vi "Path Edit.vi"() -> ()   [LabVIEW 2013]
uses:
  Global Variables.vi
panel:
  in  "Index":i32=8
  in  "Direction":u16(ring) items=["Forward", "Backward"]
  in  "Enabled":bool=TRUE
  in  "Voltage Schedule":u16(ring) items=["Constant", "Ramp", "Fn. Generator", "Formula"]
  in  "Apply to All":bool
  in  "Fill Orientation":u16(ring) items=["Horizontal", "Vertical"]
  in  "Smooth Segments":dbl=12.0
  in  "Speed Schedule":u16(ring) items=["Constant", "Ramp", "Fn. Generator", "Formula"]
  in  "Speed (µm/s)":dbl=8.0
  in  "Voltage (V)":dbl=8.0
  in  "Speed Settings":bool
  in  "Voltage Settings":bool
  in  "Fill Spacing":dbl=0.1
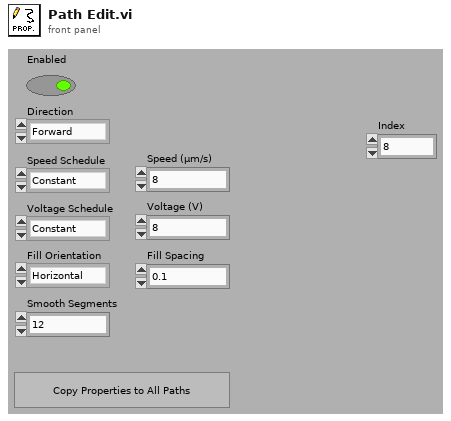
[diagram p1: front panel]
types:
  T1 = enum32{"invalid app kind", "Development System", "Run Time System", "Student Edition", "Embedded LabVIEW", "Evaluation", "Custom"}
  T2 = enum32{"Invalid", "Standard", "Closed", "Hidden", "Minimized", "Maximized"}
  T3 = cluster{"Enabled":bool, "Direction":u16, "Fill Orientation":u16, "Smooth Segments":dbl, "Fill Spacing":dbl, "Speed (µm/s)":cluster{"Schedule":u16, "Value":dbl, "Start Value":dbl, "End Value":dbl, "Min Value":dbl, "Max Value":dbl, "Duty Cycle (%)":dbl, "Signal Type":u16, "Cycle Number":dbl, "Phase (degrees)":dbl}, "Voltage (V)":cluster{"Schedule":u16, "Value":dbl, "Start Value":dbl, "End Value":dbl, "Min Value":dbl, "Max Value":dbl, "Duty Cycle (%)":dbl, "Signal Type":u16, "Cycle Number":dbl, "Phase (degrees)":dbl}}[]
  T4 = cluster{"Enabled":bool, "Direction":u16, "Fill Orientation":u16, "Smooth Segments":dbl, "Fill Spacing":dbl, "Speed (µm/s)":cluster{"Schedule":u16, "Value":dbl, "Start Value":dbl, "End Value":dbl, "Min Value":dbl, "Max Value":dbl, "Duty Cycle (%)":dbl, "Signal Type":u16, "Cycle Number":dbl, "Phase (degrees)":dbl}, "Voltage (V)":cluster{"Schedule":u16, "Value":dbl, "Start Value":dbl, "End Value":dbl, "Min Value":dbl, "Max Value":dbl, "Duty Cycle (%)":dbl, "Signal Type":u16, "Cycle Number":dbl, "Phase (degrees)":dbl}}
  T5 = cluster{"Schedule":u16, "Value":dbl, "Start Value":dbl, "End Value":dbl, "Min Value":dbl, "Max Value":dbl, "Duty Cycle (%)":dbl, "Signal Type":u16, "Cycle Number":dbl, "Phase (degrees)":dbl}
  T6 = cluster{"Schedule":u16, "Value":dbl, "Start Value":dbl, "End Value":dbl, "Min Value":dbl, "Max Value":dbl, "Duty Cycle (%)":dbl, "Speed Signal Type":u16, "Cycle Number":dbl, "Phase (degrees)":dbl}
  T7 = cluster{"Core":cluster{"Current VI Reference":refnum<vi>, "Close Panel on Exit?":bool}}
  T8 = cluster{"Current VI Reference":refnum<vi>, "Close Panel on Exit?":bool}
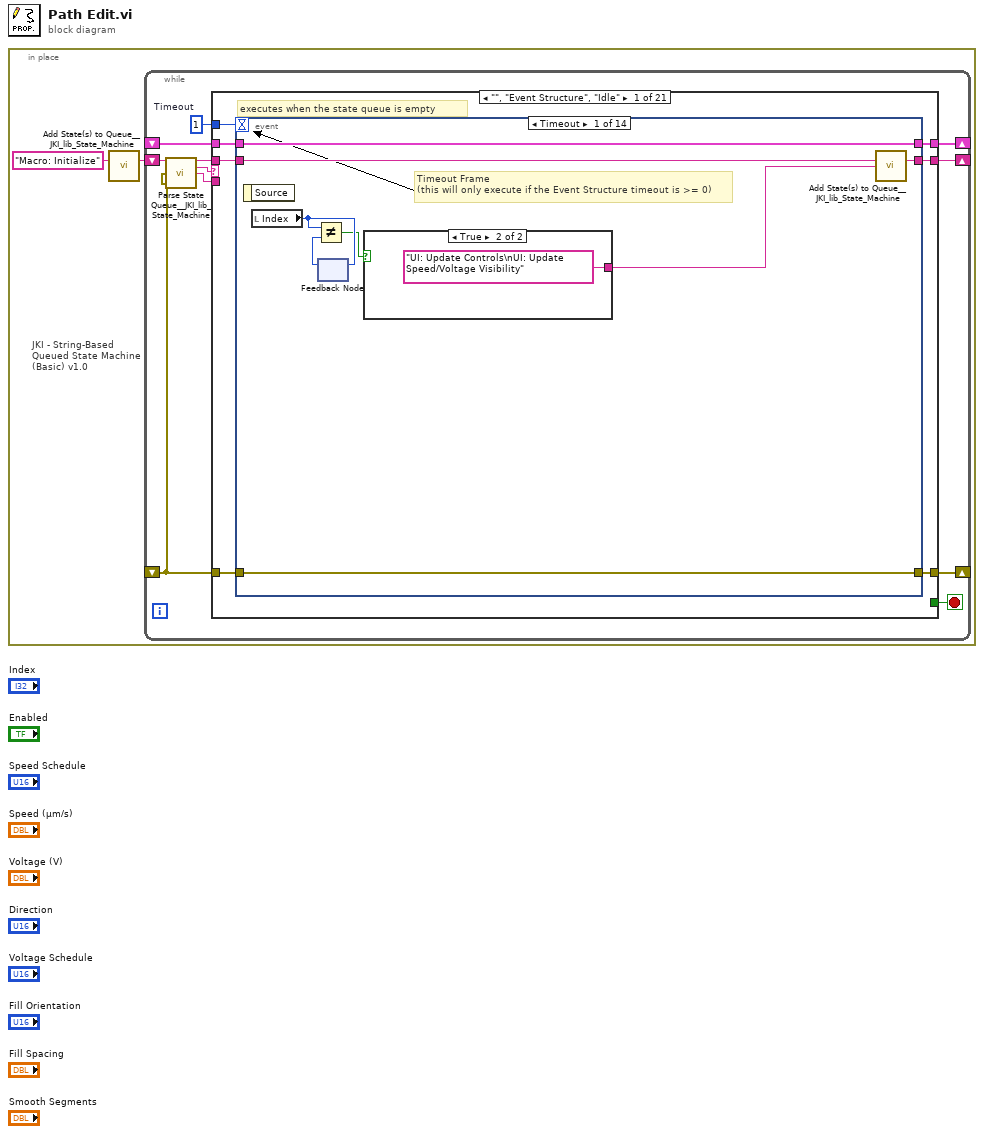
[diagram p0: block diagram]
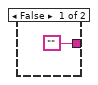
[diagram p2: hidden frame]
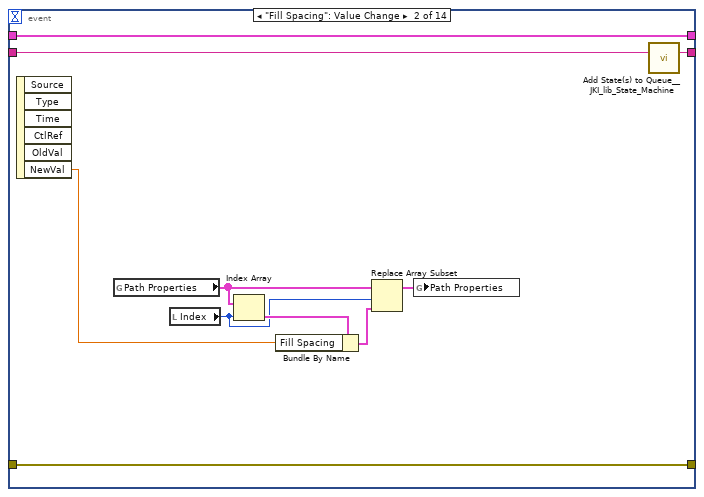
[diagram p3: hidden frame]
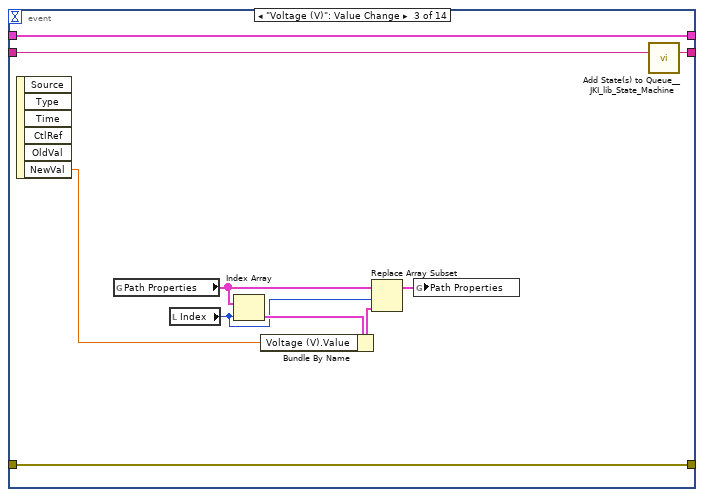
[diagram p4: hidden frame]
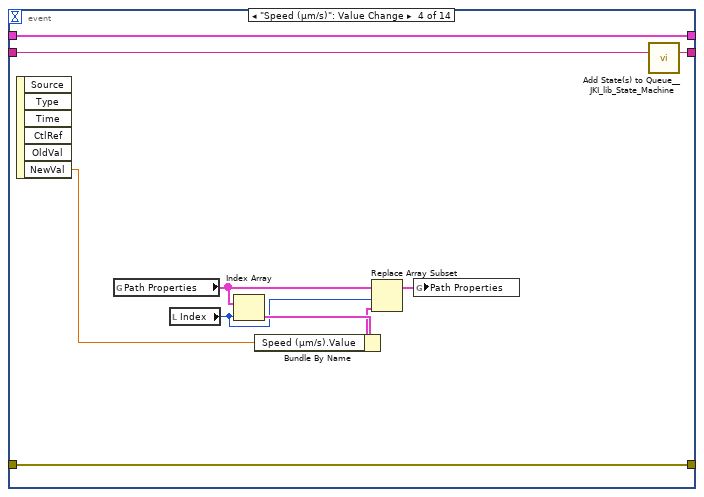
[diagram p5: hidden frame]
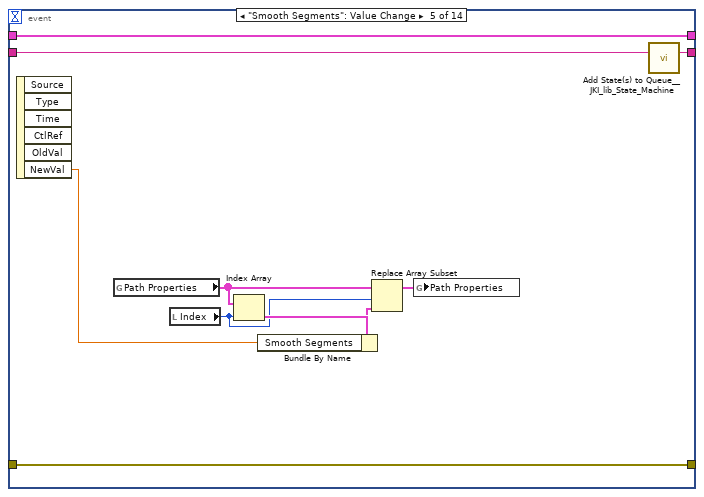
[diagram p6: hidden frame]
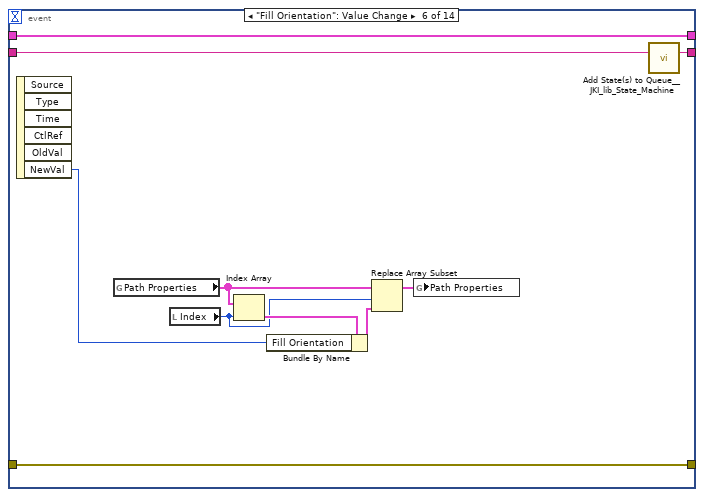
[diagram p7: hidden frame]
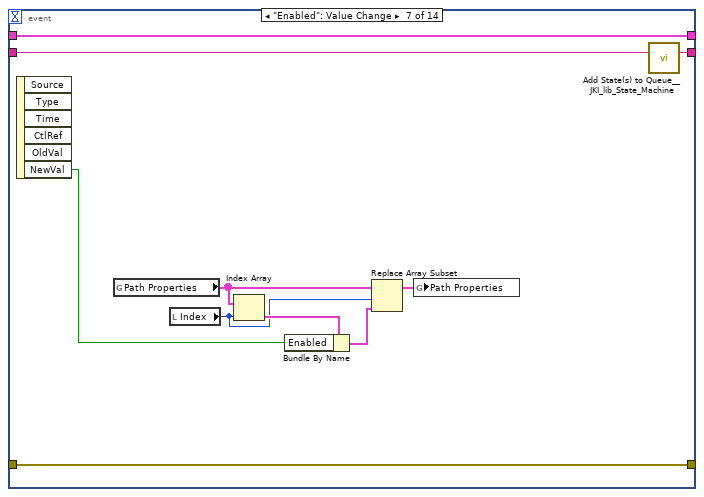
[diagram p8: hidden frame]
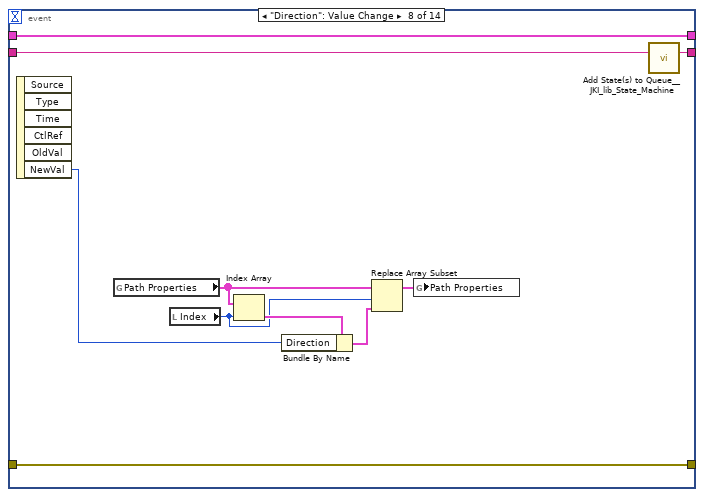
[diagram p9: hidden frame]
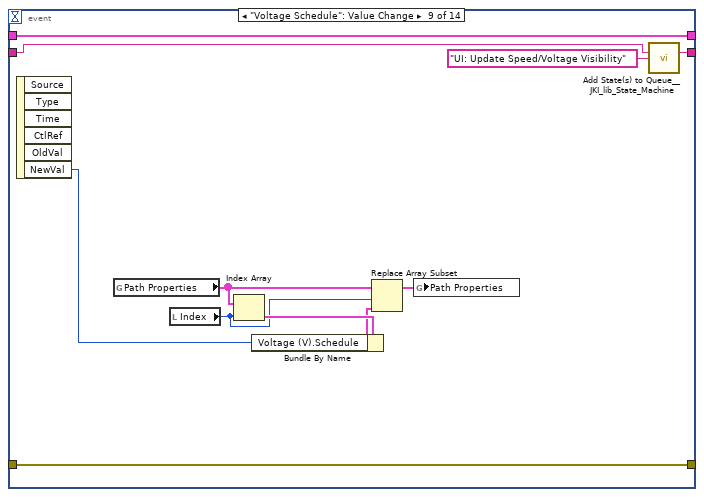
[diagram p10: hidden frame]
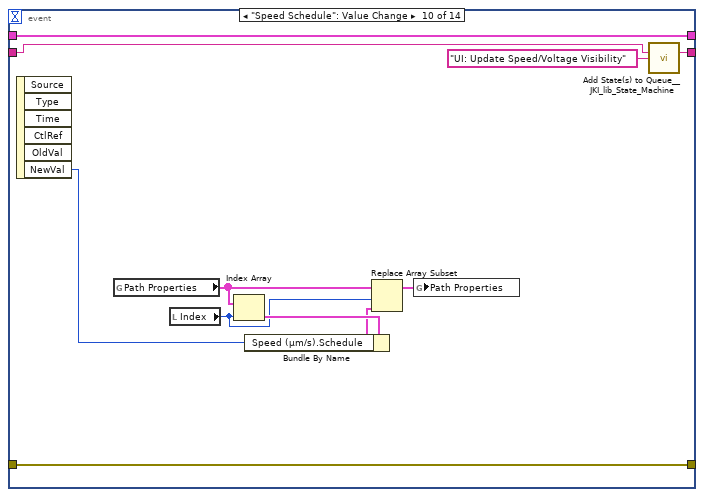
[diagram p11: hidden frame]
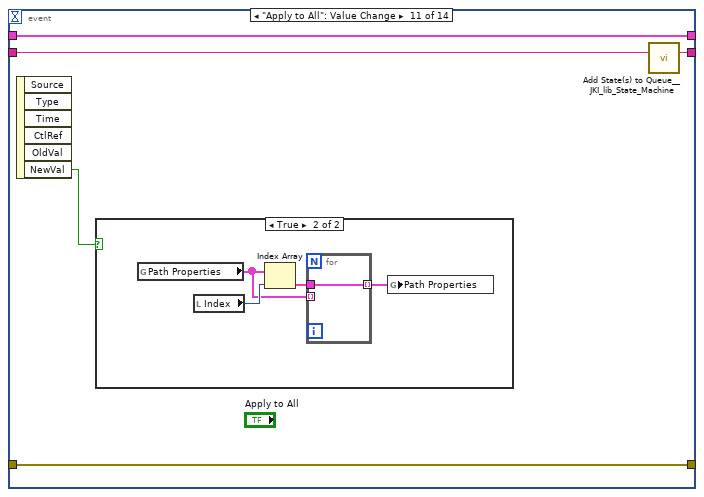
[diagram p12: hidden frame]
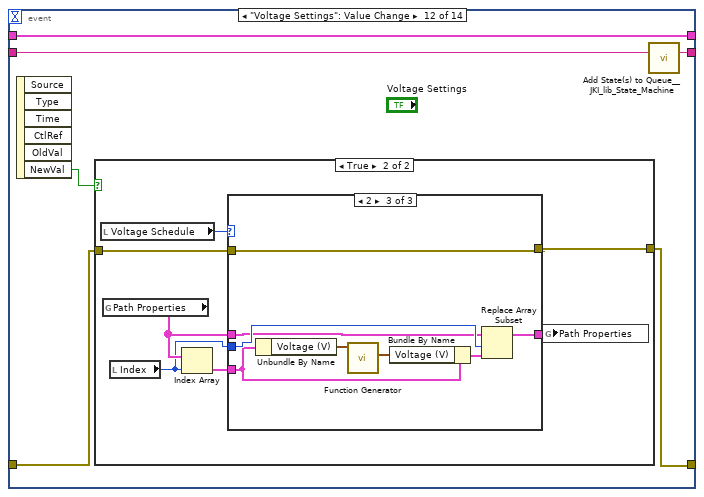
[diagram p14: hidden frame]
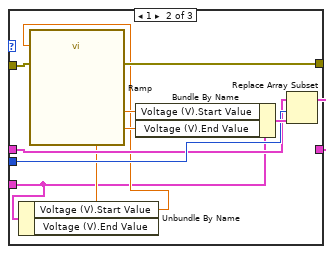
[diagram p17: hidden frame]
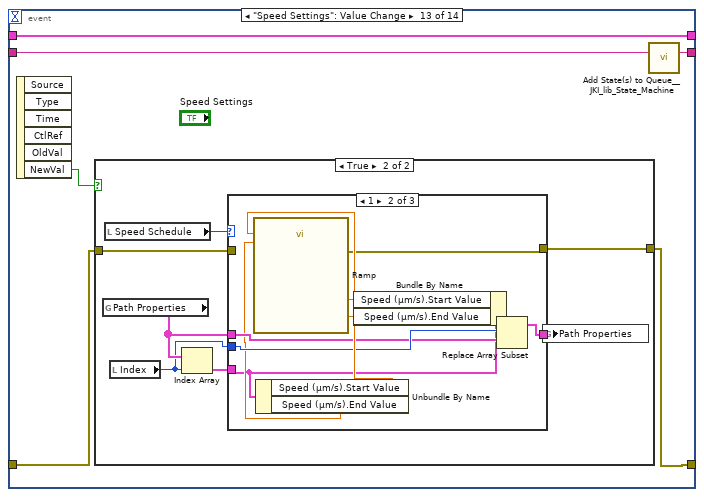
[diagram p18: hidden frame]
diagram:
  n1 = in-place {
    n2 = call <vilib>:"Add State(s) to Queue__JKI_lib_State_Machine.vi"("State(s) in (\"\")"="Macro: Initialize") -> ("States Out"=w2:string)  [unwired: 14 in]
    n3 = while "JKI - String-Based Queued State Machine (Basic) v1.0" {
      shift-right: [w6] -> _
      shift-left: _ -> [w5]
      shift-right: [w9] -> _
      shift-left: _ -> [w3]
      shift-right: [w8] -> _
      shift-left: w2 -> [w10]
      stop <- w7 stop-if-true
      w4 = 1  # Timeout
      n4 = call <vilib>:"Parse State Queue__JKI_lib_State_Machine.vi"("State Queue"=w10, "Error In (no error)"=w3) -> ("Remaining States"=w12:string, "Current State"=w13:string, "Arguments"=w11:string)  [unwired: 11 in]
      n5 = case shown="\"\", \"Event Structure\", \"Idle\"" w13 {
        selector: w13 -> [_ _ w212 _ _ _ _ _ _ _ _ _ _ _ _ _ _ _ _ _ _]
        tunnel: w12 -> [w20 w211 w216 w234 w240 w245 w249 w254 w260 w264 w268 w284 w290 w308 w319 w345 w350 w360 w364 w368 w372]
        tunnel: w11 -> [_ _ _ _ _ _ _ _ _ _ _ _ w285 _ w313 _ _ _ _ _ _]
        tunnel: w5 -> [w18 w208 w214 w230 w237 w243 w246 _ w258 w261 w266 w282 w288 w306 w315 w342 w347 w357 w361 w365 w369]
        tunnel: [w17 w209 w218 w231 errorcluster {"status"=FALSE, "code"=0, "source"=""} ("error out") w242 w247 w250 w256 w262 w265 w281 w286 w295 w316 w343 w348 w358 w362 w366 w370] -> w9
        tunnel: w3 -> [w16 w209 w217 w231 w236 w242 w247 w250 w255 w262 w265 w281 w287 w305 w317 w343 w348 w358 w362 w366 w370]
        tunnel: [w19 w210 w215 w233 w239 w244 w248 w253 w259 w263 w267 w283 w289 w307 w318 w344 w349 w359 w363 w367 w371] -> w8
        tunnel: [_ _ _ _ _ TRUE _ _ _ _ _ _ _ _ _ _ _ _ _ _ _] -> w7
        tunnel: [w15 w208 w214 w232 w237 w243 w246 w252 w258 w261 w266 w282 w288 w306 w315 w342 w347 w357 w361 w365 w369] -> w6
        tunnel: w4 -> [w14 _ _ _ _ _ _ _ _ _ _ _ _ _ _ _ _ _ _ _ _]
        frame "", "Event Structure", "Idle" {
          # "executes when the state queue is empty"
          n6 = event shown="[0] Timeout" {
            selector: _ -> [_ _ _ _ _ _ _ _ _ _ _ _ _ _]
            dyn-events: _ -> [_ _ _ _ _ _ _ _ _ _ _ _ _ _]
            timeout: w14 -> [_ _ _ _ _ _ _ _ _ _ _ _ _ _]
            tunnel: w20 -> [w28 w40 w50 w60 w70 w80 w90 w100 w111 w122 w127 w138 w173 w207]
            tunnel: [w27 w39 w49 w59 w69 w79 w89 w99 w110 w121 w126 w137 w172 w206] -> w19
            tunnel: w18 -> [w25 w38 w48 w58 w68 w78 w88 w98 w109 w120 w125 w136 w171 w204]
            tunnel: [w26 w32 w42 w52 w62 w72 w82 w92 w103 w114 w124 w134 w169 w205] -> w17
            tunnel: w16 -> [w26 w32 w42 w52 w62 w72 w82 w92 w103 w114 w124 w135 w170 w205]
            tunnel: [w25 w38 w48 w58 w68 w78 w88 w98 w109 w120 w125 w136 w171 w204] -> w15
            event Timeout {
              # "Timeout Frame\n(this will only execute if the Event Structure timeout is >= 0)"
              n7 = event-data() -> ()  [unwired: 1 in, 1 out]
              n8 = local read "Index"() -> (w23:i32)
              n9 = feedback #1() -> (w24:i32)  [unwired: 1 in]
              n10 = Not Equal?(x=w23, y=w24) -> (x != y?=w22:bool)
              n11 = feedback-in #1(w23) -> ()
              n12 = case shown="True" w22 {
                tunnel: ["" "UI: Update Controls\nUI: Update Speed/Voltage Visibility"] -> w21
                frame False {
                }
                frame True {
                }
              }
              n13 = call <vilib>:"Add State(s) to Queue__JKI_lib_State_Machine.vi"("State(s) in (\"\")"=w28, "State(s) at Back (\"\")"=w21) -> ("States Out"=w27:string)  [unwired: 13 in]
            }
            event "Fill Spacing": Value Change {
              n14 = event-data() -> ("NewVal"=w36:dbl)  [unwired: 1 in, 5 out]
              n15 = global read "Global Variables.vi" "Path Properties"() -> (w34:T3)
              n16 = local read "Index"() -> (w31:i32)
              n17 = Index Array(array=w34, index=w31) -> (element=w37:T4)
              n18 = Bundle By Name(cluster=w37, "Fill Spacing"=w36) -> (w35:T4)
              n19 = Replace Array Subset(array=w34, new element=w35, index=w31) -> (w33:T3)
              n20 = global write "Global Variables.vi" "Path Properties"(w33) -> ()
              n21 = call <vilib>:"Add State(s) to Queue__JKI_lib_State_Machine.vi"("State(s) in (\"\")"=w40) -> ("States Out"=w39:string)  [unwired: 14 in]
            }
            event "Voltage (V)": Value Change {
              n22 = event-data() -> ("NewVal"=w46:dbl)  [unwired: 1 in, 5 out]
              n23 = global read "Global Variables.vi" "Path Properties"() -> (w44:T3)
              n24 = local read "Index"() -> (w41:i32)
              n25 = Index Array(array=w44, index=w41) -> (element=w47:T4)
              n26 = Bundle By Name(cluster=w47, "Voltage (V).Value"=w46) -> (w45:T4)
              n27 = Replace Array Subset(array=w44, new element=w45, index=w41) -> (w43:T3)
              n28 = global write "Global Variables.vi" "Path Properties"(w43) -> ()
              n29 = call <vilib>:"Add State(s) to Queue__JKI_lib_State_Machine.vi"("State(s) in (\"\")"=w50) -> ("States Out"=w49:string)  [unwired: 14 in]
            }
            event "Speed (µm/s)": Value Change {
              n30 = event-data() -> ("NewVal"=w56:dbl)  [unwired: 1 in, 5 out]
              n31 = global read "Global Variables.vi" "Path Properties"() -> (w54:T3)
              n32 = local read "Index"() -> (w51:i32)
              n33 = Index Array(array=w54, index=w51) -> (element=w57:T4)
              n34 = Bundle By Name(cluster=w57, "Speed (µm/s).Value"=w56) -> (w55:T4)
              n35 = Replace Array Subset(array=w54, new element=w55, index=w51) -> (w53:T3)
              n36 = global write "Global Variables.vi" "Path Properties"(w53) -> ()
              n37 = call <vilib>:"Add State(s) to Queue__JKI_lib_State_Machine.vi"("State(s) in (\"\")"=w60) -> ("States Out"=w59:string)  [unwired: 14 in]
            }
            event "Smooth Segments": Value Change {
              n38 = event-data() -> ("NewVal"=w66:dbl)  [unwired: 1 in, 5 out]
              n39 = global read "Global Variables.vi" "Path Properties"() -> (w64:T3)
              n40 = local read "Index"() -> (w61:i32)
              n41 = Index Array(array=w64, index=w61) -> (element=w67:T4)
              n42 = Bundle By Name(cluster=w67, "Smooth Segments"=w66) -> (w65:T4)
              n43 = Replace Array Subset(array=w64, new element=w65, index=w61) -> (w63:T3)
              n44 = global write "Global Variables.vi" "Path Properties"(w63) -> ()
              n45 = call <vilib>:"Add State(s) to Queue__JKI_lib_State_Machine.vi"("State(s) in (\"\")"=w70) -> ("States Out"=w69:string)  [unwired: 14 in]
            }
            event "Fill Orientation": Value Change {
              n46 = event-data() -> ("NewVal"=w76:u16)  [unwired: 1 in, 5 out]
              n47 = global read "Global Variables.vi" "Path Properties"() -> (w74:T3)
              n48 = local read "Index"() -> (w71:i32)
              n49 = Index Array(array=w74, index=w71) -> (element=w77:T4)
              n50 = Bundle By Name(cluster=w77, "Fill Orientation"=w76) -> (w75:T4)
              n51 = Replace Array Subset(array=w74, new element=w75, index=w71) -> (w73:T3)
              n52 = global write "Global Variables.vi" "Path Properties"(w73) -> ()
              n53 = call <vilib>:"Add State(s) to Queue__JKI_lib_State_Machine.vi"("State(s) in (\"\")"=w80) -> ("States Out"=w79:string)  [unwired: 14 in]
            }
            event "Enabled": Value Change {
              n54 = event-data() -> ("NewVal"=w86:bool)  [unwired: 1 in, 5 out]
              n55 = global read "Global Variables.vi" "Path Properties"() -> (w84:T3)
              n56 = local read "Index"() -> (w81:i32)
              n57 = Index Array(array=w84, index=w81) -> (element=w87:T4)
              n58 = Bundle By Name(cluster=w87, "Enabled"=w86) -> (w85:T4)
              n59 = Replace Array Subset(array=w84, new element=w85, index=w81) -> (w83:T3)
              n60 = global write "Global Variables.vi" "Path Properties"(w83) -> ()
              n61 = call <vilib>:"Add State(s) to Queue__JKI_lib_State_Machine.vi"("State(s) in (\"\")"=w90) -> ("States Out"=w89:string)  [unwired: 14 in]
            }
            event "Direction": Value Change {
              n62 = event-data() -> ("NewVal"=w96:u16)  [unwired: 1 in, 5 out]
              n63 = global read "Global Variables.vi" "Path Properties"() -> (w94:T3)
              n64 = local read "Index"() -> (w91:i32)
              n65 = Index Array(array=w94, index=w91) -> (element=w97:T4)
              n66 = Bundle By Name(cluster=w97, "Direction"=w96) -> (w95:T4)
              n67 = Replace Array Subset(array=w94, new element=w95, index=w91) -> (w93:T3)
              n68 = global write "Global Variables.vi" "Path Properties"(w93) -> ()
              n69 = call <vilib>:"Add State(s) to Queue__JKI_lib_State_Machine.vi"("State(s) in (\"\")"=w100) -> ("States Out"=w99:string)  [unwired: 14 in]
            }
            event "Voltage Schedule": Value Change {
              n70 = event-data() -> ("NewVal"=w107:u16)  [unwired: 1 in, 5 out]
              n71 = global read "Global Variables.vi" "Path Properties"() -> (w105:T3)
              n72 = local read "Index"() -> (w101:i32)
              n73 = Index Array(array=w105, index=w101) -> (element=w108:T4)
              n74 = Bundle By Name(cluster=w108, "Voltage (V).Schedule"=w107) -> (w106:T4)
              n75 = Replace Array Subset(array=w105, new element=w106, index=w101) -> (w104:T3)
              n76 = global write "Global Variables.vi" "Path Properties"(w104) -> ()
              n77 = call <vilib>:"Add State(s) to Queue__JKI_lib_State_Machine.vi"("State(s) in (\"\")"=w111, "State(s) at Back (\"\")"="UI: Update Speed/Voltage Visibility" ("State(s) at Back (\"\")")) -> ("States Out"=w110:string)  [unwired: 13 in]
            }
            event "Speed Schedule": Value Change {
              n78 = event-data() -> ("NewVal"=w118:u16)  [unwired: 1 in, 5 out]
              n79 = global read "Global Variables.vi" "Path Properties"() -> (w116:T3)
              n80 = local read "Index"() -> (w112:i32)
              n81 = Index Array(array=w116, index=w112) -> (element=w119:T4)
              n82 = Bundle By Name(cluster=w119, "Speed (µm/s).Schedule"=w118) -> (w117:T4)
              n83 = Replace Array Subset(array=w116, new element=w117, index=w112) -> (w115:T3)
              n84 = global write "Global Variables.vi" "Path Properties"(w115) -> ()
              n85 = call <vilib>:"Add State(s) to Queue__JKI_lib_State_Machine.vi"("State(s) in (\"\")"=w122, "State(s) at Back (\"\")"="UI: Update Speed/Voltage Visibility" ("State(s) at Back (\"\")")) -> ("States Out"=w121:string)  [unwired: 13 in]
            }
            event "Apply to All": Value Change {
              n86 = event-data() -> ("NewVal"=w123:bool)  [unwired: 1 in, 5 out]
              n87 = case shown="True" w123 {
                frame False {
                }
                frame True {
                  n88 = global read "Global Variables.vi" "Path Properties"() -> (w128:T3)
                  n89 = local read "Index"() -> (w131:i32)
                  n90 = Index Array(array=w128, index=w131) -> (element=w130:T4)
                  n91 = for {
                    tunnel: w130 -> [w132]
                    tunnel: [w132] -> w129 mode=indexing
                    tunnel: w128 -> [_] mode=indexing
                  }
                  n92 = global write "Global Variables.vi" "Path Properties"(w129) -> ()
                }
              }
              n93 = call <vilib>:"Add State(s) to Queue__JKI_lib_State_Machine.vi"("State(s) in (\"\")"=w127) -> ("States Out"=w126:string)  [unwired: 14 in]
            }
            event "Voltage Settings": Value Change {
              n94 = event-data() -> ("NewVal"=w133:bool)  [unwired: 1 in, 5 out]
              n95 = case shown="True" w133 {
                tunnel: w135 -> [w139 w145]
                tunnel: [w139 w144] -> w134
                frame False {
                }
                frame True {
                  n96 = local read "Voltage Schedule"() -> (w146:u16)
                  n97 = global read "Global Variables.vi" "Path Properties"() -> (w141:T3)
                  n98 = local read "Index"() -> (w140:i32)
                  n99 = Index Array(array=w141, index=w140) -> (element=w142:T4)
                  n100 = case shown="2" w146 {
                    tunnel: w145 -> [w148 w159 w163]
                    tunnel: [w148 w152 w163] -> w144
                    tunnel: [w147 w153 w164] -> w143
                    tunnel: w142 -> [_ w149 w162]
                    tunnel: w141 -> [w147 w154 w165]
                    tunnel: w140 -> [_ w155 w166]
                    frame 0, Default {
                    }
                    frame 1 {
                      n101 = Unbundle By Name(w149) -> ("Voltage (V).Start Value"=w151:dbl, "Voltage (V).End Value"=w150:dbl)
                      n102 = call "Ramp.vi"("Start Value"=w151, "End Value"=w150, "error in (no error)"=w159) -> ("End Value"=w157:dbl, "Start Value"=w158:dbl, "error out"=w152:errorcluster)  [unwired: 13 in, 1 out]
                      n103 = Bundle By Name(cluster=w149, "Voltage (V).Start Value"=w158, "Voltage (V).End Value"=w157) -> (w156:T4)
                      n104 = Replace Array Subset(array=w154, new element=w156, index=w155) -> (w153:T3)
                    }
                    frame 2 {
                      n105 = Unbundle By Name(w162) -> ("Voltage (V)"=w160:T5)
                      n106 = call "Function Generator.vi"("Properties in"=w160) -> ("Properties out"=w161:T6)  [unwired: 9 in, 1 out]
                      n107 = Bundle By Name(cluster=w162, "Voltage (V)"=w161) -> (w167:T4)
                      n108 = Replace Array Subset(array=w165, new element=w167, index=w166) -> (w164:T3)
                    }
                  }
                  n109 = global write "Global Variables.vi" "Path Properties"(w143) -> ()
                }
              }
              n110 = call <vilib>:"Add State(s) to Queue__JKI_lib_State_Machine.vi"("State(s) in (\"\")"=w138) -> ("States Out"=w137:string)  [unwired: 14 in]
            }
            event "Speed Settings": Value Change {
              n111 = event-data() -> ("NewVal"=w168:bool)  [unwired: 1 in, 5 out]
              n112 = case shown="True" w168 {
                tunnel: w170 -> [w174 w180]
                tunnel: [w174 w179] -> w169
                frame False {
                }
                frame True {
                  n113 = global read "Global Variables.vi" "Path Properties"() -> (w176:T3)
                  n114 = local read "Speed Schedule"() -> (w181:u16)
                  n115 = local read "Index"() -> (w175:i32)
                  n116 = Index Array(array=w176, index=w175) -> (element=w177:T4)
                  n117 = case shown="1" w181 {
                    tunnel: w180 -> [w183 _ w197]
                    tunnel: [w183 w189 w197] -> w179
                    tunnel: [w182 w188 w198] -> w178
                    tunnel: w177 -> [_ w184 w196]
                    tunnel: w176 -> [w182 w186 w199]
                    tunnel: w175 -> [_ w187 w200]
                    frame 0, Default {
                    }
                    frame 1 {
                      n118 = Unbundle By Name(w184) -> ("Speed (µm/s).Start Value"=w190:dbl, "Speed (µm/s).End Value"=w185:dbl)
                      n119 = call "Ramp.vi"("Start Value"=w190, "End Value"=w185) -> ("End Value"=w192:dbl, "Start Value"=w193:dbl, "error out"=w189:errorcluster)  [unwired: 14 in, 1 out]
                      n120 = Bundle By Name(cluster=w184, "Speed (µm/s).Start Value"=w193, "Speed (µm/s).End Value"=w192) -> (w191:T4)
                      n121 = Replace Array Subset(array=w186, new element=w191, index=w187) -> (w188:T3)
                    }
                    frame 2 {
                      n122 = Unbundle By Name(w196) -> ("Speed (µm/s)"=w194:T5)
                      n123 = call "Function Generator.vi"("Properties in"=w194) -> ("Properties out"=w195:T6)  [unwired: 9 in, 1 out]
                      n124 = Bundle By Name(cluster=w196, "Speed (µm/s)"=w195) -> (w201:T4)
                      n125 = Replace Array Subset(array=w199, new element=w201, index=w200) -> (w198:T3)
                    }
                  }
                  n126 = global write "Global Variables.vi" "Path Properties"(w178) -> ()
                }
              }
              n127 = call <vilib>:"Add State(s) to Queue__JKI_lib_State_Machine.vi"("State(s) in (\"\")"=w173) -> ("States Out"=w172:string)  [unwired: 14 in]
            }
            event Panel Close? {
              # "Discard the event because we'll close the front panel ourselves in Macro: Exit"
              # "Close Panel button (pressed) Event\n(this executes Macro: Exit to terminate the VI)"
              n128 = event-data() -> ()  [unwired: 1 in, 1 out]
              n129 = event-data("Discard?"=TRUE) -> ()  [unwired: 1 in, 1 out]
              n130 = call <vilib>:"Add State(s) to Queue__JKI_lib_State_Machine.vi"("State(s) in Front (\"\")"="Macro: Exit", "State(s) in (\"\")"=w207) -> ("States Out"=w206:string)  [unwired: 13 in]
            }
          }
        }
        frame "---------- Core ----------" {
          # "Do not put any code in this frame.\n(it is a separator no-op)"
          n131 = call <vilib>:"Add State(s) to Queue__JKI_lib_State_Machine.vi"("State(s) in (\"\")"=w211) -> ("States Out"=w210:string)  [unwired: 14 in]
        }
        frame Default {
          w221 = 42 items=["No error", "Argument error", "Memory is full", "Out of zone", "End of file", "File already open", "Generic file I/O error", "File not found", "File permission error", "Disk is full", "Duplicate path", "Too many files open", "System feature not enabled", "Resource file not found", "Cannot add resource", "Resource not found", "Image not found", "Image memory error", "Pen does not exist", "Config type invalid", "Config token not found", "Config parse error", "Config memory error", "Bad external code format", "Bad external code offset", "External code not present", "Null window", "Destroy window error", "Null menu", "Print aborted", "Bad print record", "Print driver error", "Windows error during printing", "Memory error during printing", "Print dialog error", "Generic print error", "Invalid device refnum", "Device not found", "Device parameter error", "Device unit error", "Cannot open device", "Device call aborted", "Generic error", "Cancelled by user", "Object ID too low", "Object ID too high", "Object not in heap", "Unknown heap", "Unknown object (invalid DefProc)", "Unknown object (DefProc not in table)", "Message out of range", "Invalid (null) method", "Unknown message", "Manager call not supported", "Bad address", "Network operation in progress", "Network operation timed out", "Connection is busy", "Network attribute not supported", "Network error", "Address in use", "System out of memory", "Connection aborted", "Connection refused", "Not connected", "Already connected", "Connection closed", "Initialization error (interapplication manager)", "Bad occurrence", "Wait on unbound occurrence handler", "Occurrence queue overflow", "Datalog type conflict", "Unused", "Unrecognized type (interapplication manager)", "Memory corrupt", "Failed to make temporary DLL", "Old CIN version", "Drag socket not found", "Failed to load drop-object", "Failed to register OLE object", "Failed to release OLE object", "Format specifier type mismatch", "Unknown format specifier", "Too few format specifiers", "Too many format specifiers", "Scan failed", "Newer CIN version", "Error converting to variant", "Runtime menu error", "Password tampered", "Variant attribute not found", "Incompatible variant data type", "Event data is not available", "Event Store is not present", "Occurrence is not found", "Event Queue is not created", "Event info is not available", "Refnum passed is NULL", "Error retrieving Class GUID", "Error retrieving CoClass GUID", "Error retrieving TypeLib GUID.", "Bad built application magic bytes.", "Specific driver is different from the specific driver associated with the Logical Name.", "There is no session opened to the class driver.", "Max Error", "MAX - Error with config objects", "MAX - Error loading configuration", "MAX - Group not supported"]
          # "Current State"
          # "Do not delete, rename, or modify this frame.\n(this is used to capture unhandled states and typos)"
          # "Handle mistyped state name (developer tool)"
          n132 = Format Into String(format string="Software Exception: Unhandled State \"%s\"." ("message"), error in=w217, w212) -> (resulting string=w220:string, error out=w219:errorcluster)  [unwired: 1 in]
          n133 = call <vilib>:"Error Cluster From Error Code.vi"("show call chain? (False)"=TRUE, "error in (no error)"=w219, "error message (\"\")"=w220, "error code (0)"=w221) -> ("error out"=w218:errorcluster)  [unwired: 5 in]
          n134 = call <vilib>:"Add State(s) to Queue__JKI_lib_State_Machine.vi"("State(s) in (\"\")"=w216) -> ("States Out"=w215:string)  [unwired: 14 in]
        }
        frame "Initialize Core Data" {
          # "exe?"
          # "If panel starts closed or is an EXE, then close it when we exit"
          # "Do not delete, rename, or modify this frame.\n(this is used to determine panel behavior on exit)"
          n135 = control-ref of="Current VI Reference"() -> (w229:refnum<vi>)
          n136 = property class="VI"() -> ("Front Panel.Open"=w228:bool)  [unwired: 2 in, 2 out]
          n137 = property class="App"() -> ("App.Kind"=w227:T1)  [unwired: 2 in, 2 out]
          n138 = Not(x=w228) -> (.not. x?=w225:bool)
          n139 = Equal?(x=w227, y=T1."Run Time System" ("Application:Kind")) -> (x = y?=w224:bool)
          n140 = Or(x=w225, y=w224) -> (x .or. y?=w223:bool)
          n141 = Bundle By Name(cluster=w230, "Core.Current VI Reference"=w229, "Core.Close Panel on Exit?"=w223) -> (w232:T7)
          n142 = call <vilib>:"Add State(s) to Queue__JKI_lib_State_Machine.vi"("State(s) in (\"\")"=w234) -> ("States Out"=w233:string)  [unwired: 14 in]
        }
        frame "Error Handler" {
          # "Unhandled Error -- Display it"
          # "Handle any errors here.\nYou can also output any states to clean-up after errors occur"
          # "Clear error"
          n143 = call <vilib>:"General Error Handler.vi"("error in (no error)"=w236) -> ()  [unwired: 10 in, 5 out]
          n144 = call <vilib>:"Add State(s) to Queue__JKI_lib_State_Machine.vi"("State(s) in Front (\"\")"="/* Post Error States", "State(s) in (\"\")"=w240) -> ("States Out"=w239:string)  [unwired: 13 in]
        }
        frame "Exit" {
          # "Do not put any code in this frame.\n(No errors that occur here will be handled.)"
          n145 = call <vilib>:"Add State(s) to Queue__JKI_lib_State_Machine.vi"("State(s) in (\"\")"=w245) -> ("States Out"=w244:string)  [unwired: 14 in]
        }
        frame "---------- Data ----------" {
          # "Do not put any code in this frame.\n(It is a separator no-op. You can make a copy of this frame to create a new Data frame)"
          n146 = call <vilib>:"Add State(s) to Queue__JKI_lib_State_Machine.vi"("State(s) in (\"\")"=w249) -> ("States Out"=w248:string)  [unwired: 14 in]
        }
        frame "Data: Initialize" {
          w251 = T8 {"Current VI Reference"=refnum, "Close Panel on Exit?"=FALSE}  # Core
          # "Initialize the shift-register data, here.\n(data names are defined by what you wire into the bundle function)"
          n147 = Bundle("Core"=w251) -> (w252:T7)  [unwired: 1 in]
          n148 = call <vilib>:"Add State(s) to Queue__JKI_lib_State_Machine.vi"("State(s) in (\"\")"=w254) -> ("States Out"=w253:string)  [unwired: 14 in]
        }
        frame "Data: Cleanup" {
          # "Cleanup any data and references, here.\n(this is called automatically, by the Macro: Exit)"
          n149 = Unbundle By Name(w258) -> ("Core.Current VI Reference"=w257:refnum<vi>)
          n150 = Close Reference(reference=w257, error in (no error)=w255) -> (error out=w256:errorcluster)
          n151 = call <vilib>:"Add State(s) to Queue__JKI_lib_State_Machine.vi"("State(s) in (\"\")"=w260) -> ("States Out"=w259:string)  [unwired: 14 in]
        }
        frame "---------- UI ----------" {
          # "Do not put any code in this frame.\n(It is a separator no-op. You can make a copy of this frame to create a new UI frame)"
          n152 = call <vilib>:"Add State(s) to Queue__JKI_lib_State_Machine.vi"("State(s) in (\"\")"=w264) -> ("States Out"=w263:string)  [unwired: 14 in]
        }
        frame "UI: Initialize" {
          # "Initialize the User Interface, here.\n(this is called automatically, by the Macro: Init)"
          n153 = call <vilib>:"Add State(s) to Queue__JKI_lib_State_Machine.vi"("State(s) in (\"\")"=w268) -> ("States Out"=w267:string)  [unwired: 14 in]
        }
        frame "UI: Update Controls" {
          n154 = global read "Global Variables.vi" "Path Properties"() -> (w269:T3)
          n155 = local read "Index"() -> (w273:i32)
          n156 = Index Array(array=w269, index=w273) -> (element=w272:T4)
          n157 = Unbundle By Name(w272) -> ("Enabled"=w274:bool, "Direction"=w275:u16, "Fill Orientation"=w276:u16, "Smooth Segments"=w277:dbl, "Fill Spacing"=w278:dbl, "Speed (µm/s).Schedule"=w271:u16, "Speed (µm/s).Value"=w279:dbl, "Voltage (V).Schedule"=w270:u16, "Voltage (V).Value"=w280:dbl)
          n158 = local write "Enabled"(w274) -> ()
          n159 = local write "Direction"(w275) -> ()
          n160 = local write "Fill Orientation"(w276) -> ()
          n161 = local write "Smooth Segments"(w277) -> ()
          n162 = local write "Fill Spacing"(w278) -> ()
          n163 = local write "Speed Schedule"(w271) -> ()
          n164 = local write "Speed (µm/s)"(w279) -> ()
          n165 = local write "Voltage Schedule"(w270) -> ()
          n166 = local write "Voltage (V)"(w280) -> ()
          n167 = call <vilib>:"Add State(s) to Queue__JKI_lib_State_Machine.vi"("State(s) in (\"\")"=w284) -> ("States Out"=w283:string)  [unwired: 14 in]
        }
        frame "UI: Cursor Set" {
          # "Argument"
          # "Set and Unset Cursor Busy.\n(Usage: \"UI: Cursor Set >> Busy|Idle\")"
          n168 = case shown="\"Idle\", Default" w285 {
            tunnel: w287 -> [w292 w294]
            tunnel: [w291 w293] -> w286
            frame "Idle", Default {
              n169 = call <vilib>:"Unset Busy.vi"("error in (no error)"=w292) -> ("error out"=w291:errorcluster)  [unwired: 10 in]
            }
            frame "Busy" {
              n170 = call <vilib>:"Set Busy.vi"("error in (no error)"=w294) -> ("error out"=w293:errorcluster)  [unwired: 9 in, 1 out]
            }
          }
          n171 = call <vilib>:"Add State(s) to Queue__JKI_lib_State_Machine.vi"("State(s) in (\"\")"=w290) -> ("States Out"=w289:string)  [unwired: 14 in]
        }
        frame "UI: Update Speed/Voltage Visibility" {
          n172 = local read "Voltage Schedule"() -> (w304:u16)
          n173 = case shown="0" w304 {
            tunnel: [TRUE FALSE] -> w300
            frame 0 {
            }
            frame 1, Default {
            }
          }
          n174 = local read "Speed Schedule"() -> (w303:u16)
          n175 = property on="Voltage (V)" class="DigNum (strict)"(error in=w305, "Visible"=w300) -> (error out=w301:errorcluster)  [unwired: 1 in, 1 out]
          n176 = case shown="0" w303 {
            tunnel: [TRUE FALSE] -> w296
            frame 0 {
            }
            frame 1, Default {
            }
          }
          n177 = Not(x=w300) -> (.not. x?=w299:bool)
          n178 = property on="Voltage Settings" class="Bool"(error in=w301, "Visible"=w299) -> (error out=w298:errorcluster)  [unwired: 1 in, 1 out]
          n179 = property on="Speed (µm/s)" class="DigNum (strict)"(error in=w298, "Visible"=w296) -> (error out=w297:errorcluster)  [unwired: 1 in, 1 out]
          n180 = Not(x=w296) -> (.not. x?=w302:bool)
          n181 = property on="Speed Settings" class="Bool"(error in=w297, "Visible"=w302) -> (error out=w295:errorcluster)  [unwired: 1 in, 1 out]
          n182 = call <vilib>:"Add State(s) to Queue__JKI_lib_State_Machine.vi"("State(s) in (\"\")"=w308) -> ("States Out"=w307:string)  [unwired: 14 in]
        }
        frame "UI: Front Panel State" {
          # "Argument"
          # "Set Front Panel Open or Closed\n(Usage: \"UI: Front Panel State >> Open|Close\")"
          n183 = Unbundle By Name(w315) -> ("Core.Current VI Reference"=w314:refnum<vi>)
          n184 = case shown="\"Open\", Default" w313 {
            tunnel: w317 -> [w323 w336]
            tunnel: [w325 w337] -> w316
            tunnel: w314 -> [w324 w334]
            frame "Open", Default {
              n185 = property class="VI"(reference=w324, error in=w323) -> (reference out=w321:refnum<vi>, error out=w322:errorcluster, "Front Panel.Open"=w320:bool)
              n186 = case shown="False" w320 {
                tunnel: [w328 w331] -> w325
                tunnel: w322 -> [w327 w331]
                tunnel: w321 -> [w326 _]
                frame False {
                  n187 = invoke class="VI" method="FP.Open"(reference=w326, error in=w327, "Activate"=TRUE, "State"=T2."Standard") -> (error out=w328:errorcluster)  [unwired: 1 in, 4 out]
                }
                frame True {
                }
              }
            }
            frame "Close" {
              n188 = property class="VI"(reference=w334, error in=w336) -> (reference out=w333:refnum<vi>, error out=w335:errorcluster, "Front Panel.Open"=w332:bool)
              n189 = case shown="True" w332 {
                tunnel: [w338 w341] -> w337
                tunnel: w335 -> [w338 w340]
                tunnel: w333 -> [_ w339]
                frame False {
                }
                frame True {
                  n190 = invoke class="VI" method="FP.Close"(reference=w339, error in=w340) -> (error out=w341:errorcluster)  [unwired: 1 in, 2 out]
                }
              }
            }
          }
          n191 = call <vilib>:"Add State(s) to Queue__JKI_lib_State_Machine.vi"("State(s) in (\"\")"=w319) -> ("States Out"=w318:string)  [unwired: 14 in]
        }
        frame "---------- Macro ----------" {
          # "Do not put any code in this frame.\n(It is a separator no-op. You can make a copy of this frame to create a new Macro frame)"
          n192 = call <vilib>:"Add State(s) to Queue__JKI_lib_State_Machine.vi"("State(s) in (\"\")"=w345) -> ("States Out"=w344:string)  [unwired: 14 in]
        }
        frame "Macro: Initialize" {
          w346 = "Data: Initialize\nInitialize Core Data\nUI: Initialize\nUI: Update Controls\nUI: Update Speed/Voltage Visibility\nUI: Front Panel State >> Close"  # Data: Initialize Initialize Core Data UI: Initialize UI: Update Controls UI: Update Speed/Voltage Visibility UI: Front Panel State >> Close
          # "Initialization Macro\n(This is called once, when the VI starts)"
          n193 = call <vilib>:"Add State(s) to Queue__JKI_lib_State_Machine.vi"("State(s) in Front (\"\")"=w346, "State(s) in (\"\")"=w350) -> ("States Out"=w349:string)  [unwired: 13 in]
        }
        frame "Macro: Exit" {
          # "Exit Macro\n(This is called once, when the VI exits)"
          n194 = Unbundle By Name(w357) -> ("Core.Close Panel on Exit?"=w356:bool)
          n195 = Select(t="UI: Front Panel State >> Close", s=w356, f="") -> (s? t:f=w353:string)
          n196 = call <vilib>:"Add State(s) to Queue__JKI_lib_State_Machine.vi"("State(s) in (\"\")"=w353, "State(s) at Back (\"\")"="Data: Cleanup\nExit") -> ("States Out"=w351:string)  [unwired: 13 in]
          n197 = call <vilib>:"Add State(s) to Queue__JKI_lib_State_Machine.vi"("State(s) in Front (\"\")"=w351, "State(s) in (\"\")"=w360) -> ("States Out"=w359:string)  [unwired: 13 in]
        }
        frame "---------- New Category ----------" {
          # "Template Separator\n(You can make a copy of, or modify, this frame)"
          n198 = call <vilib>:"Add State(s) to Queue__JKI_lib_State_Machine.vi"("State(s) in (\"\")"=w364) -> ("States Out"=w363:string)  [unwired: 14 in]
        }
        frame "New Category: 1" {
          # "Your code here.\n(You can make a copy of, or modify, this frame)"
          n199 = call <vilib>:"Add State(s) to Queue__JKI_lib_State_Machine.vi"("State(s) in (\"\")"=w368) -> ("States Out"=w367:string)  [unwired: 14 in]
        }
        frame "New Category: 2" {
          # "Your code here.\n(You can make a copy of, or modify, this frame)"
          n200 = call <vilib>:"Add State(s) to Queue__JKI_lib_State_Machine.vi"("State(s) in (\"\")"=w372) -> ("States Out"=w371:string)  [unwired: 14 in]
        }
      }
    }
  }
